vi "Start Function Blocks.vi"(8 "错误输入（无错误）":errorcluster, 11 "子面板数组":refnum<vi>[](array[refnum])) -> (0 "错误输出":errorcluster)   [LabVIEW 2018, in "MainInterface.lvlib"]
uses:
  MainInterface.lvlib
  ModuleInterface/ModuleInterface.lvlib
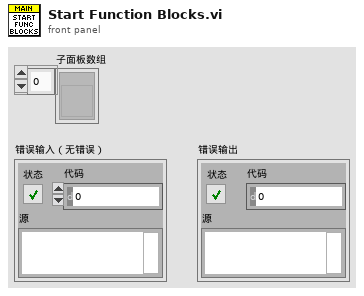
[diagram p1: front panel]
types:
  T1 = typedef "ModuleInterface.lvlib/ModuleDefinition.ctl" = cluster{"模块名称":string, "项定义":T2[]}
  T2 = typedef "ModuleInterface.lvlib/FunctionItem.ctl" = cluster{"项名":string, "符号图形路径":path}
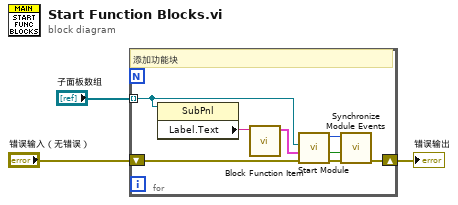
[diagram p0: block diagram]
diagram:
  n1 = for {
    shift-right: [w6] -> w2
    shift-left: "错误输入（无错误）" -> [w11]
    tunnel: "子面板数组" -> [w5] mode=indexing
    # "添加功能块"
    n2 = property class="SubPnl"(reference=w5) -> ("Label.Text"=w4:string)  [unwired: 1 in, 2 out]
    n3 = call "Block Function Item.vi"("模块名称"=w4) -> ("模块定义"=w10:T1)  [unwired: 10 in]
    n4 = call "Start Module.vi"("error in"=w11, "模块定义"=w10, "rSubPanel"=w5) -> ("error out"=w9:errorcluster, "Wait for Event Sync?"=w8:bool, "Module ID"=w7:i32)  [unwired: 5 in, 1 out]
    n5 = call "Synchronize Module Events.vi"("error in"=w9, "Wait for Event Sync?"=w8, "Module ID in"=w7) -> ("error out"=w6:errorcluster)  [unwired: 7 in, 1 out]
  }
  "错误输出" <- w2
